vi "Tracepoint_FlushToDisk.vi"(6 "out of disk space":bool=TRUE, 7 "Qbus":refnum<class "Qbus.lvclass">, 8 "error in (no error)":errorcluster, 9 "file path":path, 10 "wrote to disk":bool=TRUE, 11 "data":variant) -> (0 "error out":errorcluster)   [LabVIEW 2017, in "FileManager.lvlib"]
uses:
  <vilib>/addons/InsightCM/Devices/Shared/Common/FileManager/FileManager.lvlib
  <vilib>/addons/Qbus/Qbus.lvclass
  <vilib>/addons/TraceLogger/TraceLogger.lvlib
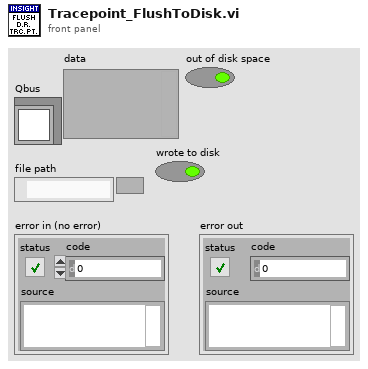
[diagram p1: front panel]
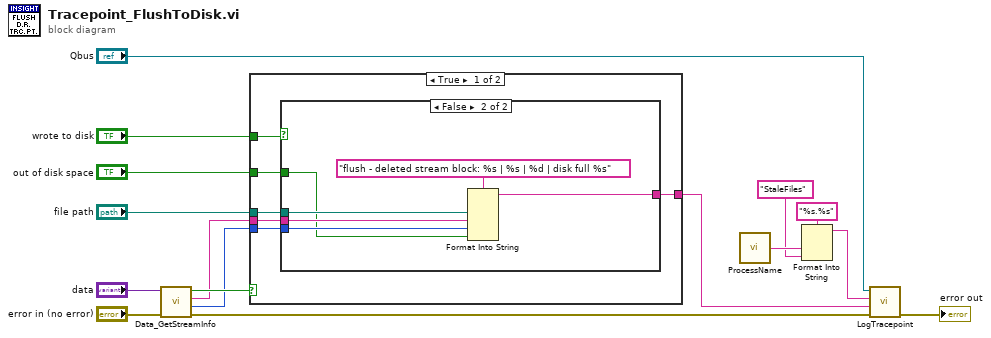
[diagram p0: block diagram]
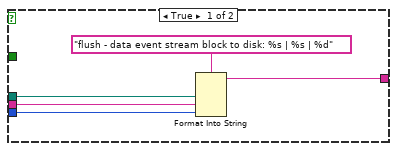
[diagram p2: hidden frame]
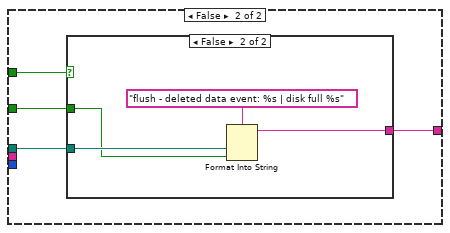
[diagram p3: hidden frame]
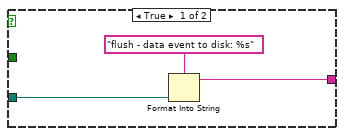
[diagram p4: hidden frame]
diagram:
  n1 = call <vilib>:"Data_GetStreamInfo.vi"("error in (no error)"="error in (no error)", "data"="data") -> ("error out"=w6:errorcluster, "block"=w11:i32, "stream Id"=w12:string, "found"=w13:bool)  [unwired: 6 in]
  n2 = case shown="True" w13 {
    tunnel: "file path" -> [w22 w37]
    tunnel: [w21 w36] -> w4
    tunnel: w12 -> [w20 _]
    tunnel: w11 -> [w19 _]
    tunnel: "wrote to disk" -> [w18 w35]
    tunnel: "out of disk space" -> [w17 w34]
    frame True {
      n3 = case shown="False" w18 {
        tunnel: w22 -> [w27 w33]
        tunnel: [w26 w32] -> w21
        tunnel: w20 -> [w24 w30]
        tunnel: w19 -> [w23 w29]
        tunnel: w17 -> [_ w28]
        frame True {
          n4 = Format Into String(format string="flush - data event stream block to disk: %s | %s | %d", w27, w24, w23) -> (resulting string=w26:string)  [unwired: 2 in, 1 out]
        }
        frame False {
          n5 = Format Into String(format string="flush - deleted stream block: %s | %s | %d | disk full %s", w33, w30, w29, w28) -> (resulting string=w32:string)  [unwired: 2 in, 1 out]
        }
      }
    }
    frame False {
      n6 = case shown="False" w35 {
        tunnel: w37 -> [w40 w44]
        tunnel: [w39 w43] -> w36
        tunnel: w34 -> [_ w41]
        frame True {
          n7 = Format Into String(format string="flush - data event to disk: %s", w40) -> (resulting string=w39:string)  [unwired: 2 in, 1 out]
        }
        frame False {
          n8 = Format Into String(format string="flush - deleted data event: %s | disk full %s", w44, w41) -> (resulting string=w43:string)  [unwired: 2 in, 1 out]
        }
      }
    }
  }
  n9 = call <vilib>:"ProcessName.vi"() -> ("process name"=w10:string)  [unwired: 5 in]
  n10 = Format Into String(format string="%s.%s", w10, "StaleFiles" ("tracepoint")) -> (resulting string=w3:string)  [unwired: 2 in, 1 out]
  n11 = call <vilib>:"LogTracepoint.vi"("error in (no error)"=w6, "log string"=w4, "tracepoint"=w3, "qbus in"="Qbus") -> ("error out"=→"error out":errorcluster)  [unwired: 6 in, 1 out]
